vi "FINAL PROJECT.vi"() -> ()   [LabVIEW 2017]
uses:
  <instrlib>/Keysight E36300 Series/Keysight E36300 Series.lvlib
panel:
  in  "LOW VOLTAGE":dbl
  in  "Channel (1) 3":string="1"
  in  "HIGH VOLTAGE":dbl
  in  "Channel (1) 2":string="1"
  in  "VISA resource name 3":refnum<visa-resource-name>
  out "?":dbl[](array[numeric]) format="%.3g"
  out "?":dbl[](array[numeric]) format="%.3g"
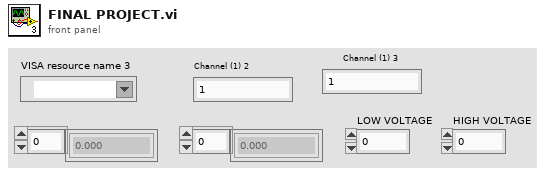
[diagram p1: front panel]
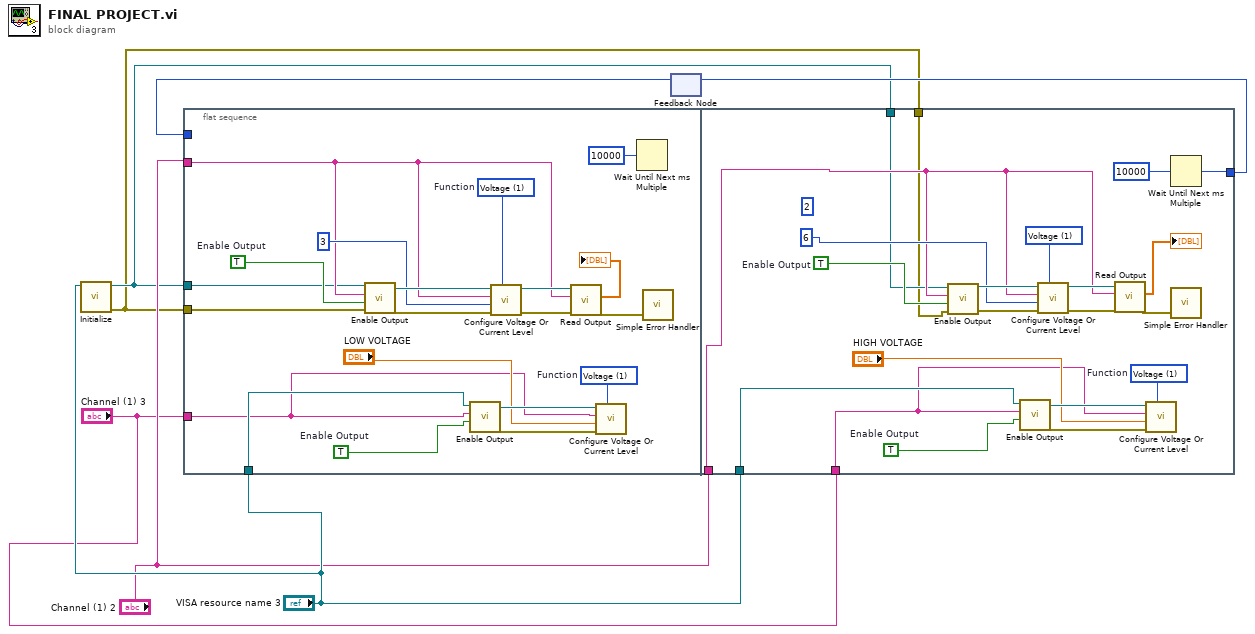
[diagram p0: block diagram]
diagram:
  n1 = call <instrlib>:"Initialize.vi"("VISA resource name"="VISA resource name 3") -> ("error out"=w1:errorcluster, "VISA resource name out"=w2:refnum<visa-resource-name>)  [unwired: 9 in]
  n2 = flat-sequence {
    tunnel: w5 -> [_]
    tunnel: "VISA resource name 3" -> [w12]
    tunnel: "Channel (1) 2" -> [w19]
    tunnel: "Channel (1) 3" -> [w10]
    tunnel: w1 -> [w9]
    tunnel: w2 -> [w8]
    tunnel: [w47] -> w7
    tunnel: "VISA resource name 3" -> [w31]
    tunnel: "Channel (1) 2" -> [w37]
    tunnel: "Channel (1) 3" -> [w28]
    tunnel: w2 -> [w30]
    tunnel: w1 -> [w29]
    frame #0 {
      w13 = TRUE  # Enable Output
      w14 = 1 items=["Current", "Voltage"]  # Function
      w24 = 1 items=["Current", "Voltage"]  # Function
      w18 = TRUE  # Enable Output
      n3 = call <instrlib>:"Enable Output.vi"("error in (no error)"=w9, "Enable Output (F: Disable)"=w18, "Channel (1)"=w19, "VISA resource name"=w8) -> ("error out"=w25:errorcluster, "VISA resource name out"=w26:refnum<visa-resource-name>)  [unwired: 6 in]
      n4 = call <instrlib>:"Enable Output.vi"("Enable Output (F: Disable)"=w13, "Channel (1)"=w10, "VISA resource name"=w12) -> ("error out"=w15:errorcluster, "VISA resource name out"=w16:refnum<visa-resource-name>)  [unwired: 7 in]
      n5 = call <instrlib>:"Configure Voltage Or Current Level.vi"("Function (0 : Current)"=w24, "error in (no error)"=w25, "Voltage Or Current Level (1)"=u32 3 ("millisecond multiple"), "Channel (1)"=w19, "VISA resource name"=w26) -> ("error out"=w20:errorcluster, "VISA resource name out"=w21:refnum<visa-resource-name>)  [unwired: 5 in]
      n6 = call <instrlib>:"Read Output.vi"("error in (no error)"=w20, "Channel (1)"=w19, "VISA resource name"=w21) -> ("error out"=w23:errorcluster, "Actual Voltage Level (V)"=→"?":dbl[])  [unwired: 5 in, 2 out]
      n7 = call <instrlib>:"Configure Voltage Or Current Level.vi"("Function (0 : Current)"=w14, "error in (no error)"=w15, "Voltage Or Current Level (1)"="LOW VOLTAGE", "Channel (1)"=w10, "VISA resource name"=w16) -> ()  [unwired: 5 in, 2 out]
      n8 = Wait Until Next ms Multiple(millisecond multiple=u32 10000) -> ()  [unwired: 1 out]
      n9 = call <vilib>:"Simple Error Handler.vi"("error in (no error)"=w23) -> ()  [unwired: 4 in, 5 out]
    }
    frame #1 {
      w33 = TRUE  # Enable Output
      w34 = 1 items=["Current", "Voltage"]  # Function
      (unwired) u32 2 ("millisecond multiple")
      w43 = 1 items=["Current", "Voltage"]
      w45 = TRUE  # Enable Output
      n10 = call <instrlib>:"Enable Output.vi"("error in (no error)"=w29, "Enable Output (F: Disable)"=w45, "Channel (1)"=w37, "VISA resource name"=w30) -> ("error out"=w44:errorcluster, "VISA resource name out"=w46:refnum<visa-resource-name>)  [unwired: 6 in]
      n11 = call <instrlib>:"Enable Output.vi"("Enable Output (F: Disable)"=w33, "Channel (1)"=w28, "VISA resource name"=w31) -> ("error out"=w35:errorcluster, "VISA resource name out"=w36:refnum<visa-resource-name>)  [unwired: 7 in]
      n12 = call <instrlib>:"Configure Voltage Or Current Level.vi"("Function (0 : Current)"=w43, "error in (no error)"=w44, "Voltage Or Current Level (1)"=u32 6 ("millisecond multiple"), "Channel (1)"=w37, "VISA resource name"=w46) -> ("error out"=w39:errorcluster, "VISA resource name out"=w40:refnum<visa-resource-name>)  [unwired: 5 in]
      n13 = call <instrlib>:"Read Output.vi"("error in (no error)"=w39, "Channel (1)"=w37, "VISA resource name"=w40) -> ("error out"=w42:errorcluster, "Actual Voltage Level (V)"=→"?":dbl[])  [unwired: 5 in, 2 out]
      n14 = call <instrlib>:"Configure Voltage Or Current Level.vi"("Function (0 : Current)"=w34, "error in (no error)"=w35, "Voltage Or Current Level (1)"="HIGH VOLTAGE", "Channel (1)"=w28, "VISA resource name"=w36) -> ()  [unwired: 5 in, 2 out]
      n15 = Wait Until Next ms Multiple(millisecond multiple=u32 10000) -> (millisecond timer value=w47:u32)
      n16 = call <vilib>:"Simple Error Handler.vi"("error in (no error)"=w42) -> ()  [unwired: 4 in, 5 out]
    }
  }
  n17 = feedback #1() -> (w5:u32)  [unwired: 1 in]
  n18 = feedback-in #1(w7) -> ()
